vi "LogData.vi"() -> ()   [LabVIEW 2017]
panel:
  in  "LogData":dbl[](array[numeric])=[0.0, 0.0, 0.0, 0.0, 0.0]
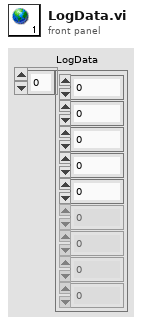
[diagram p1: front panel]
diagram:
